vi "Expt1_MT PSK Transceiver_Updated.vi"(0 "Message Symbols":i32=1000, 5 "Eb/N0, dB":dbl(slide)=40.0 scale=0.0..80.0, 7 "TX Filter":T1(ring)=enum."Root Raised Cos", 9 "Reset":bool=TRUE, 14 "?":T2(tab)=enum."Constellation (RX output)") -> (3 "PSK System Parameters":T5={"samples per symbol (16)"=4, "symbol map"=[0.7071067811865476+0.7071067811865475i, -0.7071067811865475+0.7071067811865476i, 0.7071067811865474-0.7071067811865477i, -0.7071067811865477-0.7071067811865475i], "differential PSK"=enum."disable", "PSK type"=0} {"PSK type" items=["normal", "shifted", "offset"]; "symbol map" format="%.3f"}, 4 "Output Complex Waveform":cluster{"t0":dbl, "dt":dbl, "Values":cdb[]} {"Values" format="%.3f"; "dt" format="%^.2e"; "t0" format="%.4f"}, 6 "Transmitted  Bits":i8[](array[numeric]), 8 "Received Bits":i8[](array[numeric]), 10 "Bit Error Rate":dbl format="%.4e", 13 "Last Sync Found Index":dbl format="%.4f", 15 "Error Out":errorcluster)   [LabVIEW 2020]
doc: "This example demonstrates generation and analysis of PSK modulated signals. You can specify transmit filter parameters, Eb/No, and frequency offset. This example demonstrates programming techniques for resetting the transmitter in cases where the receiver (demodulator) lock is lost. You can see the results of the demodulation on an eye-diagram plot, and perform measurements such as bit error rate."
uses:
  <vilib>/addons/Modulation/Digital/Support/Controls/PSK System Parameters.ctl
  <vilib>/addons/Modulation/Digital/Support/Common/Validators/mod_AWGN Validate.vi
  <vilib>/addons/Modulation/Analog/support/mod_Set Error Source.vi
  <vilib>/addons/Modulation/Digital/Impairments/subVIs/mod_createSeeds.vi
  <vilib>/addons/Modulation/Digital/Impairments/subVIs/mod_IQ Impairments Gain Imbalance.vi
  <vilib>/addons/Modulation/Digital/Impairments/subVIs/mod_IQ Impairments Quadrature Skew.vi
  <vilib>/addons/Modulation/Digital/Impairments/subVIs/mod_IQ Impairments Axis Shear.vi
  <vilib>/addons/Modulation/Digital/Impairments/subVIs/mod_IQ Impairments DC Offset.vi
  <vilib>/addons/Modulation/Digital/Impairments/subVIs/mod_IQ Impairments Frequency Offset.vi
  <vilib>/addons/Modulation/Digital/Support/Common/Validators/mod_Validate Samples Per Symbol.vi
  <vilib>/addons/Modulation/Analog/support/Validators/mod_Validate Complex Waveform.vi
  <vilib>/Analysis/5stat.llb/RMS.vi
  <vilib>/Analysis/5stat.llb/RMS (DBL).vi
  <vilib>/addons/Modulation/Digital/Support/Common/mod_Apply Frequency Offset.vi
  <vilib>/addons/Modulation/Analog/support/Validators/mod_WFErrorHandler.vi
  <vilib>/addons/Modulation/Digital/Support/Common/mod_Apply Frequency Offset (Internal).vi
  <vilib>/addons/Modulation/Digital/General/subVIs/mod_Generate Bits PN Sequence.vi
  <vilib>/Analysis/1siggen.llb/Gaussian White Noise (obs 90).vi
  <vilib>/addons/Modulation/Digital/Support/Common/Validators/mod_IQ Impairments Validate.vi
  <vilib>/addons/Modulation/Digital/Demodulation/MT EbN0 Calculation(PSK).vi
  <vilib>/addons/Modulation/Digital/General/MT Format Eye Diagram (complex).vi
  <vilib>/addons/Modulation/Digital/Demodulation/MT Calculate BER After Trigger (PN Sequence).vi
  <vilib>/addons/Modulation/niDMT.lvlib
  <vilib>/addons/Modulation/niAMT.lvlib
panel:
  out "Estimated Eb/N0(dB)":dbl
  out "Frequency Offset, Hz":dbl=0.0014081098665354938 format="%.2f"
  in  "Frequency Offset, Hz":dbl(slide) scale=-1000.0..1000.0
  in  "Symbol Rate":dbl=100000.0 step=1000.0 format="%.2p"
  in  "M-PSK":enum16{"2", "4", "8", "16", "32", "64"}(ring)=enum."4"
  out "Modulation Error Ratio, dB":dbl format="%.2f"
  out "BER Trigger Found":bool
  in  "Stop":bool
  out "TX Symbols":T3(graph)={{"1/x"=0.0, 1e-05, [], 1}, []}
  out "FFT Magnitude Spectrum":cluster{dbl, dbl, dbl[]}(graph)={-199899.99999999997, 99.99999999999999, []}
  out "Constellation graph":T4(graph)
  out "RX Symbols":T3(graph)={{"1/x"=0.0, 1e-05, [], 1}, []}
  in  "autoscale":bool
  out "Constellation Graph":T4(graph)
  in  "Display I/Q":enum16{"I", "Q"}(ring)=enum."Q"
  out "Eye Diagram":cluster{"t0":dbl, "dt":dbl, "Y":dbl[]}[](graph)
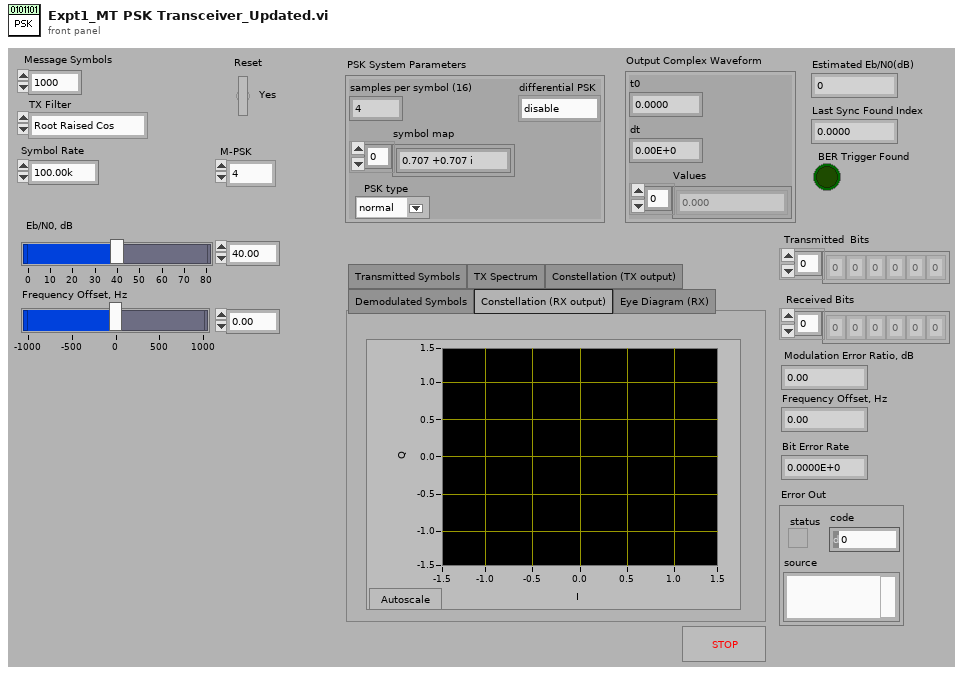
[diagram p1: front panel]
types:
  T1 = enum16{"none", "Raised Cosine", "Root Raised Cos", "Gaussian"}
  T2 = enum32{"Transmitted Symbols", "TX Spectrum", "Constellation (TX output)", "Demodulated Symbols", "Constellation (RX output)", "Eye Diagram (RX)"}
  T3 = cluster{cluster{"1/x":dbl, dbl, i8[], i32}, i32[][]}
  T4 = cluster{"Decimated Array":dbl[], "Decimated Array":dbl[]}[]
  T5 = typedef "niDMT.lvlib/PSK System Parameters.ctl" = cluster{"samples per symbol (16)":i32, "symbol map":cdb[], "differential PSK":enum16{"disable", "enable"}, "PSK type":u16}
  T6 = cluster{"expected sync location (symbols)":i32, "sync sequence":cdb[], "sync location uncertainty (symbols)":i32, "sync indent (symbols)":i32}
  T7 = cluster{"TX Filter":enum16{"none", "Raised Cosine", "Root Raised Cos", "Gaussian"}, "filter parameter":dbl, "filter length":i32}
  T8 = cluster{"M-PSK (4)":i32, "differential PSK":enum16{"disable", "enable"}, "PSK type":u16}
  T9 = cluster{"# Guard Bits":i32, "# Sync Bits":i32, "# Message Bits":i32, "PN sequence order":i32}
  T10 = cluster{"Output Bit Stream":i8[], " # bits per symbol":i32, "Sync (Bits)":i8[], "Sync (Symbols)":cdb[], "pulse shaping filter coefficients":dbl[], "matched filter coefficients":dbl[], "PSK system parameters":T5}
  T11 = typedef "niAMT.lvlib/Complex Data Waveform.ctl" = cluster{"t0":dbl, "dt":dbl, "Y":cdb[]}
  T12 = cluster{"frequency offset (Hz)":dbl, "frequency drift (Hz)":dbl, "phase offset (deg)":dbl}
  T13 = cluster{"constellation":dbl[], "oversampled data":dbl[]}[]
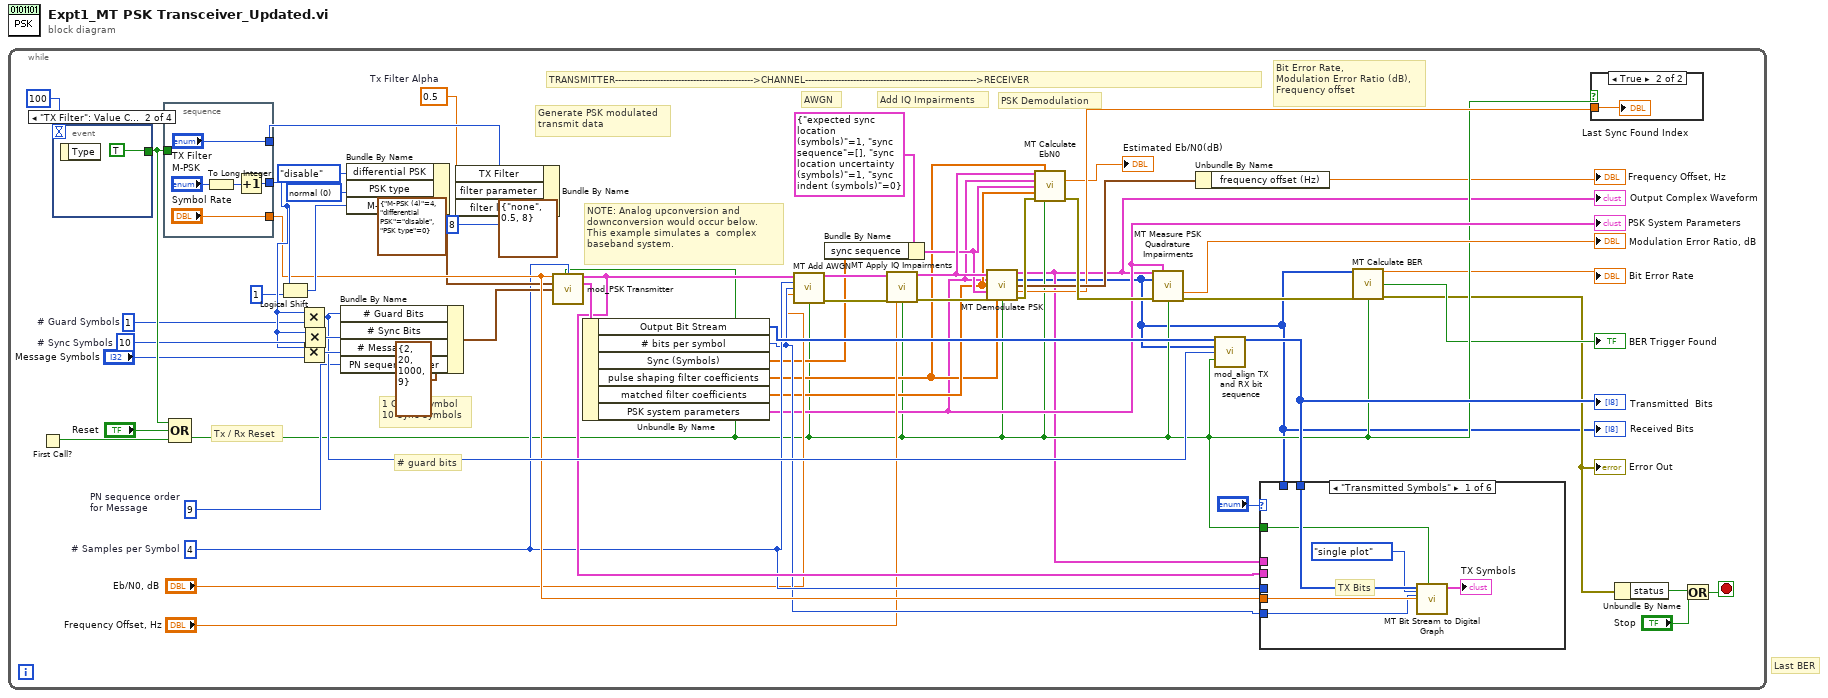
[diagram p0: block diagram]
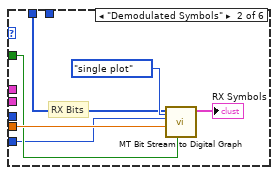
[diagram p2: hidden frame]
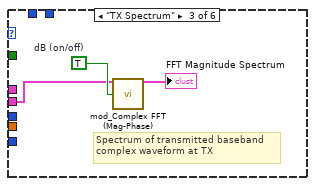
[diagram p3: hidden frame]
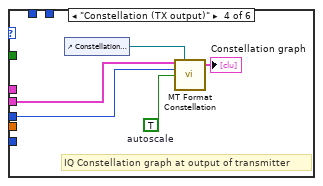
[diagram p4: hidden frame]
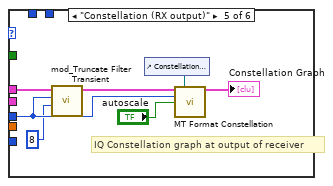
[diagram p5: hidden frame]
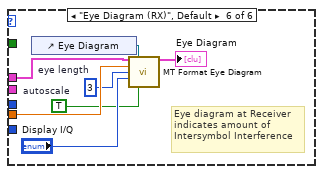
[diagram p6: hidden frame]
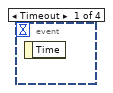
[diagram p8: hidden frame]
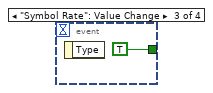
[diagram p9: hidden frame]
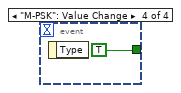
[diagram p10: hidden frame]
diagram:
  # "Last BER"
  n1 = while {
    stop <- w45 stop-if-true
    w36 = 9  # PN sequence order for Message
    w38 = 0.5  # Tx Filter Alpha
    w40 = u16 0 items=["normal", "shifted", "offset"] ("PSK type")
    w26 = 4  # # Samples per Symbol
    w54 = 10  # # Sync Symbols
    w48 = 1  # # Guard Symbols
    # "Bit Error Rate,\nModulation Error Ratio (dB),\nFrequency offset"
    # "Tx / Rx Reset"
    # "1 Guard Symbol\n10 Sync Symbols"
    # "# guard bits"
    # "Generate PSK modulated\ntransmit data"
    # "PSK Demodulation"
    # "Add IQ Impairments"
    # "AWGN"
    # "TRANSMITTER---------------------------------------------->CHANNEL--------------------------------------------------------->RECEIVER"
    # "NOTE: Analog upconversion and\ndownconversion would occur below.\nThis example simulates a  complex \nbaseband system."
    n2 = First Call?() -> (First Call?: T/F=w59:bool)
    n3 = event shown="[1] \"TX Filter\": Value Change" {
      selector: _ -> [_ _ _ _]
      dyn-events: _ -> [_ _ _ _]
      timeout: 100 -> [_ _ _ _]
      tunnel: [_ TRUE TRUE TRUE] -> w56
      event Timeout {
        n4 = event-data() -> ()  [unwired: 1 in, 1 out]
      }
      event "TX Filter": Value Change {
        n5 = event-data() -> ()  [unwired: 1 in, 1 out]
      }
      event "Symbol Rate": Value Change {
        n6 = event-data() -> ()  [unwired: 1 in, 1 out]
      }
      event "M-PSK": Value Change {
        n7 = event-data() -> ()  [unwired: 1 in, 1 out]
      }
    }
    n8 = stacked-sequence {
      tunnel: w56 -> [_]
      tunnel: ["TX Filter"] -> w52
      tunnel: [w63] -> w49
      tunnel: ["Symbol Rate"] -> w34
      frame #0 {
        n9 = To Long Integer(number="M-PSK") -> (32bit integer=w65:i32)
        n10 = Increment(x=w65) -> (x+1=w63:i32)
      }
    }
    n11 = Compound Arithmetic op=OR(w56, "Reset", w59) -> (w8:bool)
    n12 = Logical Shift(y=w49, x=1) -> (x << y=w44:i32)
    n13 = Multiply(x=w49, y=w48) -> (x*y=w47:i32)
    n14 = Multiply(x=w49, y="Message Symbols") -> (x*y=w50:i32)
    n15 = Multiply(x=w49, y=w54) -> (x*y=w53:i32)
    n16 = Bundle By Name(cluster=T9 {"# Guard Bits"=2, "# Sync Bits"=20, "# Message Bits"=1000, "PN sequence order"=9} ("Message"), "# Guard Bits"=w47, "# Sync Bits"=w53, "# Message Bits"=w50, "PN sequence order"=w36) -> (w32:T9)
    n17 = Bundle By Name(cluster=T8 {"M-PSK (4)"=4, "differential PSK"=enum."disable", "PSK type"=0} ("PSK"), "differential PSK"=enum16{"disable", "enable"}."disable", "PSK type"=w40, "M-PSK (4)"=w44) -> (w33:T8)
    n18 = Bundle By Name(cluster=T7 {"TX Filter"=enum."none", "filter parameter"=0.5, "filter length"=8} ("System Filter"), "TX Filter"=w52, "filter parameter"=w38, "filter length"=8) -> ()  [unwired: 1 out]
    n19 = call <vilib>:"mod_PSK Transmitter.vi"("Symbol Rate, Hz"=w34, "Reset?"=w8, "# Samples per Symbol"=w26, "PSK"=w33, "Message"=w32) -> ("Output Complex Waveform"=w30:cluster{"t0":dbl, "dt":dbl, "Y":cdb[]}, "Signal Description"=w31:T10)  [unwired: 8 in, 1 out]
    n20 = Unbundle By Name(w31) -> ("Output Bit Stream"=w27:i8[], "# bits per symbol"=w25:i32, "Sync (Symbols)"=w23:cdb[], "pulse shaping filter coefficients"=w16:dbl[], "matched filter coefficients"=w18:dbl[], "PSK system parameters"=w12:T5)
    "PSK System Parameters" <- w12
    n21 = call <vilib>:"MT Add AWGN.vi"("input complex waveform"=w30, "samples per symbol (16)"=w26, "bits per symbol (1)"=w25, "Eb/N0 (10 dB)"="Eb/N0, dB", "reset? (T)"=w8) -> ("output complex waveform"=w29:T11, "error out"=w28:errorcluster)  [unwired: 8 in, 1 out]
    n22 = Bundle By Name(cluster=T6 {"expected sync location (symbols)"=1, "sync sequence"=[], "sync location uncertainty (symbols)"=1, "sync indent (symbols)"=0} ("synchronization parameters"), "sync sequence"=w23) -> (w19:T6)
    n23 = call <vilib>:"MT Apply IQ Impairments.vi"("input complex waveform"=w29, "error in (no error)"=w28, "frequency offset (Hz)"="Frequency Offset, Hz", "reset? (T)"=w8) -> ("output complex waveform"=w20:T11, "error out"=w21:errorcluster)  [unwired: 10 in]
    n24 = call <vilib>:"MT Demodulate PSK.vi"("input complex waveform"=w20, "PSK system parameters"=w12, "matched filter coefficients"=w18, "synchronization parameters"=w19, "error in (no error)"=w21, "pulse shaping filter coefficients"=w16, "reset? (T)"=w8) -> ("recovered complex waveform"=w4:T11, "output bit stream"=w2:i8[], "measurements"=w14:T12, "sync found index (symbols)"=w13:dbl, "error out"=w17:errorcluster)  [unwired: 4 in]
    "Output Complex Waveform" <- w4
    "Received Bits" <- w2
    n25 = call-poly <vilib>:"MT Calculate EbN0.vi"("Recieved waveform"=w20, "pulse shaping filter coefficients"=w16, "PSK system parameters"=w12, "synchronization parameters"=w19, "matched filter coefficients"=w18, "error in (no error)"=w17, "reset? (T)"=w8) -> ("Eb/N0(dB)"=→"Estimated Eb/N0(dB)":dbl, "error out"=w15:errorcluster)  [unwired: 6 in, 1 out]
    n26 = call <vilib>:"MT Measure PSK Quadrature Impairments.vi"("recovered complex waveform"=w4, "PSK system parameters"=w12, "input bit stream"=w2, "error in (no error)"=w15, "reset? (T)"=w8) -> ("modulation error ratio (dB)"=→"Modulation Error Ratio, dB":dbl, "error out"=w9:errorcluster)  [unwired: 3 in, 6 out]
    n27 = Unbundle By Name(w14) -> ("frequency offset (Hz)"=→"Frequency Offset, Hz":dbl)
    n28 = call <vilib>:"mod_align TX and RX bit sequence.vi"("TX Bit Sequence"=w27, "RX Bit Sequence"=w2, "# Bits removed"=w47, "Reset"=w8) -> ("Aligned array"=w46:i8[])  [unwired: 11 in]
    "Transmitted  Bits" <- w46
    n29 = case shown="\"Transmitted Symbols\"" "?" {
      tunnel: w34 -> [w72 w78 _ _ _ w100]
      tunnel: w26 -> [_ _ _ w83 w90 _]
      tunnel: w46 -> [w71 _ _ _ _ _]
      tunnel: w8 -> [w70 w75 _ _ _ _]
      tunnel: w30 -> [_ _ w79 w82 _ _]
      tunnel: w25 -> [w67 w73 _ _ _ _]
      tunnel: w2 -> [_ w74 _ _ _ _]
      tunnel: w4 -> [_ _ _ _ w87 w94]
      frame "Transmitted Symbols" {
        # "TX Bits"
        n30 = call <vilib>:"MT Bit Stream to Digital Graph.vi"("Reset (F)"=w70, "Format"=enum16{"single plot", "plot per bit"}."single plot", "Symbol Rate (Hz)"=w72, "bits per symbol"=w67, "Bit Stream"=w71) -> ("Digital Waveform Graph"=→"TX Symbols":T3)  [unwired: 6 in]
      }
      frame "Demodulated Symbols" {
        # "RX Bits"
        n31 = call <vilib>:"MT Bit Stream to Digital Graph.vi"("Reset (F)"=w75, "Format"=enum16{"single plot", "plot per bit"}."single plot", "Symbol Rate (Hz)"=w78, "bits per symbol"=w73, "Bit Stream"=w74) -> ("Digital Waveform Graph"=→"RX Symbols":T3)  [unwired: 6 in]
      }
      frame "TX Spectrum" {
        w80 = TRUE  # dB (on/off)
        # "Spectrum of transmitted baseband\ncomplex waveform at TX"
        n32 = call <vilib>:"mod_Complex FFT (Mag-Phase).vi"("Input Data Waveform"=w79, "dB (on/off)"=w80) -> ("Magnitude"=→"FFT Magnitude Spectrum":cluster{"f0":dbl, "df":dbl, "Y":dbl[]})  [unwired: 12 in, 1 out]
      }
      frame "Constellation (TX output)" {
        w86 = TRUE  # autoscale
        # "IQ Constellation graph at output of transmitter"
        n33 = control-ref of="Constellation graph"() -> (w84:refnum<vi>)
        n34 = call <vilib>:"MT Format Constellation.vi"("waveform"=w82, "constellation reference"=w84, "samples per symbol"=w83, "autoscale"=w86) -> ("constellation graph"=→"Constellation graph":T13)  [unwired: 10 in, 1 out]
      }
      frame "Constellation (RX output)" {
        # "IQ Constellation graph at output of receiver"
        n35 = call <vilib>:"mod_Truncate Filter Transient.vi"("filter length (sym)"=8, "samples/symbol"=w90, "input complex waveform"=w87) -> ("output complex waveform"=w91:T11)  [unwired: 8 in]
        n36 = control-ref of="Constellation Graph"() -> (w92:refnum<vi>)
        n37 = call <vilib>:"MT Format Constellation.vi"("waveform"=w91, "constellation reference"=w92, "samples per symbol"=w90, "autoscale"="autoscale") -> ("constellation graph"=→"Constellation Graph":T13)  [unwired: 10 in, 1 out]
      }
      frame "Eye Diagram (RX)", Default {
        w97 = TRUE  # autoscale
        w99 = 3  # eye length
        # "Eye diagram at Receiver\nindicates amount of\nIntersymbol Interference"
        n38 = control-ref of="Eye Diagram"() -> (w95:refnum<vi>)
        n39 = call-poly <vilib>:"MT Format Eye Diagram.vi"("waveform"=w94, "eye diagram reference"=w95, "symbol rate (Hz)"=w100, "eye length"=w99, "I/Q (I)"="Display I/Q", "autoscale"=w97) -> ("eye diagram"=→"Eye Diagram":cluster{"t0":dbl, "dt":dbl, "Y":dbl[]}[])  [unwired: 8 in, 1 out]
      }
    }
    n40 = call-poly <vilib>:"MT Calculate BER.vi"("input bit stream"=w2, "error in (no error)"=w9, "reset? (T)"=w8) -> ("BER"=→"Bit Error Rate":dbl, "trigger found?"=→"BER Trigger Found":bool, "error out"=w5:errorcluster)  [unwired: 8 in, 2 out]
    "Error Out" <- w5
    n41 = case shown="True" w8 {
      tunnel: w13 -> [_ w101]
      frame False {
      }
      frame True {
        "Last Sync Found Index" <- w101
      }
    }
    n42 = Unbundle By Name(w5) -> ("status"=w3:bool)
    n43 = Or(x=w3, y="Stop") -> (x .or. y?=w45:bool)
  }
